vi "SetCellPos.vi"(8 "error in (no error)":errorcluster, 10 "Position":T1, 11 "SnakeBodyCell in":refnum<class "SnakeBodyCell.lvclass">) -> (0 "error out":errorcluster, 3 "SnakeBodyCell out":refnum<class "SnakeBodyCell.lvclass">)   [LabVIEW 2018, in "SnakeBodyCell.lvclass"]
uses:
  SnakeBodyCell.lvclass
  Typedefs/XYposition.ctl
  SnakeBodyCell.lvclass/SnakeBodyCell.ctl
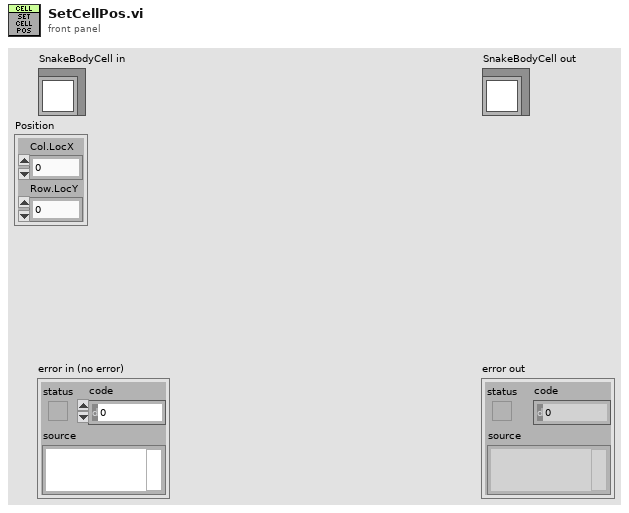
[diagram p1: front panel]
types:
  T1 = typedef "XYposition.ctl" = cluster{"Col.LocX":i32, "Row.LocY":i32}
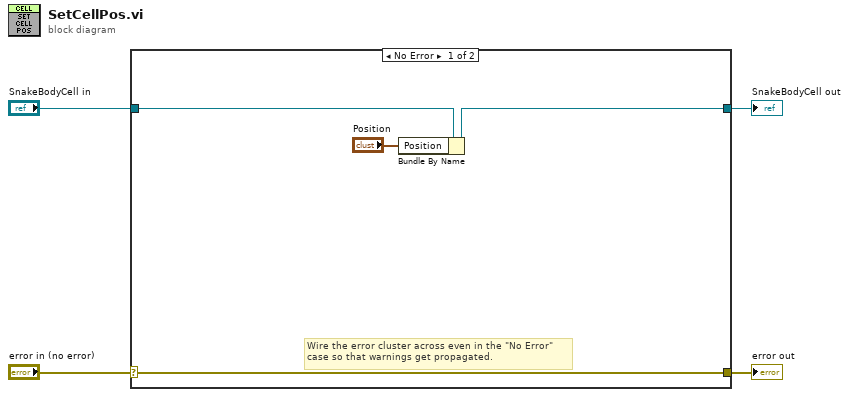
[diagram p0: block diagram]
diagram:
  n1 = case shown="No Error" "error in (no error)" {
    selector: "error in (no error)" -> [w7 w10]
    tunnel: [w7 w10] -> w3
    tunnel: [w6 w9] -> w1
    tunnel: "SnakeBodyCell in" -> [w8 w9]
    frame No Error {
      # "Wire the error cluster across even in the \"No Error\"\ncase so that warnings get propagated."
      n2 = Bundle By Name(cluster=w8, "Position"="Position") -> (w6:refnum<class "SnakeBodyCell.lvclass">)
    }
    frame Error {
    }
  }
  "error out" <- w3
  "SnakeBodyCell out" <- w1
